vi "_RT_Pub command_ping.vi"(7 "Loop Times":i32=20, 8 "error in (no error)":errorcluster, 11 "PCIP String":string="100.100.0.11") -> (0 "error out":errorcluster={"status"=TRUE, "code"=5004, "source"="Ping TimeOut"})   [LabVIEW 2018]
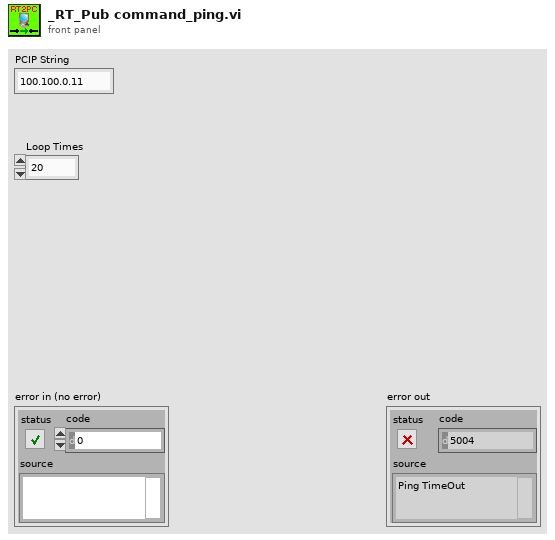
[diagram p1: front panel]
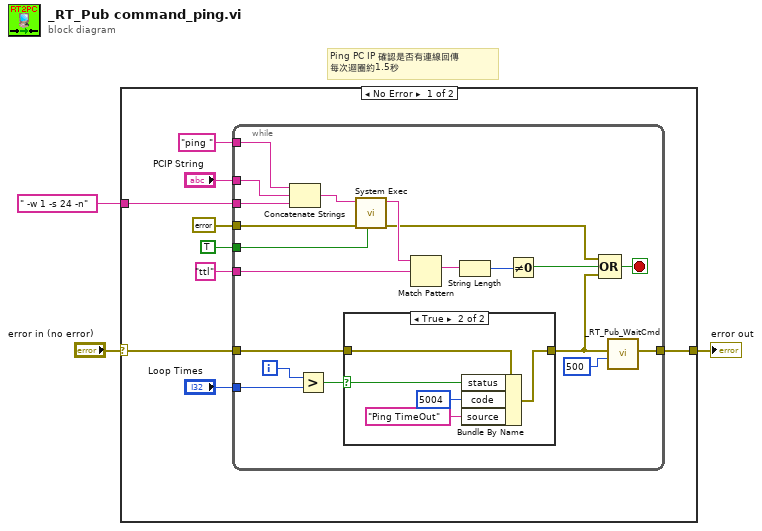
[diagram p0: block diagram]
diagram:
  # "Ping PC IP 確認是否有連線回傳\n每次迴圈約1.5秒"
  n1 = case shown="No Error" "error in (no error)" {
    selector: "error in (no error)" -> [w8 w39]
    tunnel: [w10 w39] -> w3
    tunnel: " -w 1 -s 24 -n" -> [w4 _]
    frame No Error {
      n2 = while {
        tunnel: w8 -> [w30]
        tunnel: [w14] -> w10
        tunnel: "ping " -> [w27]
        tunnel: "PCIP String" -> [w26]
        tunnel: "Loop Times" -> [w25]
        tunnel: errorcluster {"status"=FALSE, "code"=0, "source"=""} ("error in (no error)") -> [w19]
        tunnel: TRUE ("run minimized? (F)") -> [w18]
        tunnel: "ttl" ("regular expression") -> [w17]
        tunnel: w4 -> [w16]
        i -> [w32]
        stop <- w20 stop-if-true
        n3 = Concatenate Strings(w27, w26, w16) -> (w28:string)
        n4 = Greater?(x=w32, y=w25) -> (0:w31:bool)
        n5 = case shown="True" w31 {
          selector: w31 -> [_ w37]
          tunnel: w30 -> [w33 w38]
          tunnel: [w33 w34] -> w15
          frame False {
          }
          frame True {
            n6 = Bundle By Name(cluster=w38, "status"=w37, "code"=5004, "source"="Ping TimeOut") -> (w34:errorcluster)
          }
        }
        n7 = call <vilib>:"System Exec.vi"("run minimized? (F)"=w18, "error in (no error)"=w19, "command line"=w28) -> ("error out"=w22:errorcluster, "standard output"=w24:string)  [unwired: 5 in, 2 out]
        n8 = Match Pattern(string=w24, regular expression=w17) -> (match substring=w23:string)  [unwired: 1 in, 3 out]
        n9 = String Length(string=w23) -> (length=w29:i32)
        n10 = Not Equal To 0?(x=w29) -> (x != 0?=w21:bool)
        n11 = Compound Arithmetic op=OR(w22, w21, w15) -> (w20:bool)
        n12 = call "_RT_Pub_WaitCmd.vi"("milliseconds to wait"=u32 500, "error in (no error)"=w15) -> ("error out"=w14:errorcluster)  [unwired: 9 in]
      }
    }
    frame Error {
    }
  }
  "error out" <- w3
